vi "demo.vi"() -> ()   [LabVIEW 2012]
uses:
  Machine Opt.ctl
panel:
  in  "停止":bool
  out "Relay":bool[](array[boolean])
  in  "Machine Opt":T1=enum."送电启动"
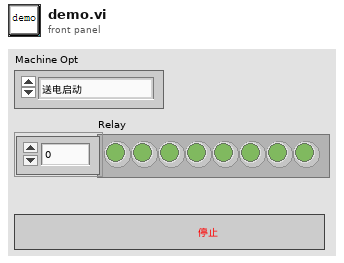
[diagram p1: front panel]
types:
  T1 = typedef "Machine Opt.ctl" = enum16{"初始化", "送电启动", "送电关闭", "液压站启动", "液压站停止", "润滑启动", "润滑停止", "冷却启动", "冷却停止", "快进启动", "快进停止", "工进启动", "工进停止", "快退启动", "快退停止", "报警启动", "报警停止"}
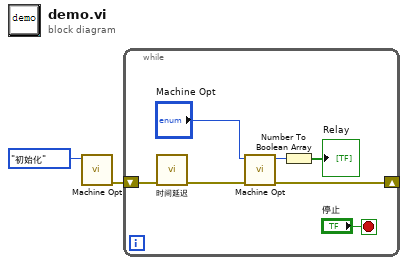
[diagram p0: block diagram]
diagram:
  n1 = call "Machine Opt.vi"("Machine Opt"=Machine_Opt."初始化") -> ("error out"=w1:errorcluster)  [unwired: 9 in, 1 out]
  n2 = while {
    shift-right: [w6] -> _
    shift-left: w1 -> [w9]
    stop <- "停止" stop-if-true
    n3 = call "时间延迟"("error in (no error)"=w9) -> ("error out"=w8:errorcluster)  [unwired: 10 in]
    n4 = call "Machine Opt.vi"("error in (no error)"=w8, "Machine Opt"="Machine Opt") -> ("error out"=w6:errorcluster, "Output(U8)"=w5:u8)  [unwired: 8 in]
    n5 = Number To Boolean Array(number=w5) -> (Boolean array=→"Relay":bool[])
  }
